vi "Load Settings from XML.vi"(8 "error in (no error)":errorcluster, 11 "Settings in":T1={"Logging Configuration"={"Log File Base Path"=path "", "NbrIma"=1}, "camera"={"Camera.lvclass"=refnum, "InClusTiming 2"={"Pixelclock"=24, "Exposure"=46.39115, "ExposureTimeBase"=2, "Framerate"=14.99615, "TriggerMode"=0}, "ROI"={"PosX"=0, "PosY"=0, "Width"=0, "Height"=0}, "File Path Control"=path "", "mirror.lvclass"=refnum}} {"camera"."InClusTiming 2"."TriggerMode" items=["Auto", "Software", "External sequence start ", "External exposure control"]; "camera"."InClusTiming 2"."ExposureTimeBase" items=["nanoseconds", "microseconds", "milliseconds"]; "camera"."InClusTiming 2"."Pixelclock" min=1 max=400 step=1 scale=0.05915..400.0 scale format="%#.3g"; "camera"."InClusTiming 2"."Framerate" min=0.05915 max=2000.0 step=1.0 scale=0.05915..100.0 scale format="%#.3g"; "camera"."InClusTiming 2"."Exposure" min=0.05915 max=2000.0 step=1.0 scale=0.05915..100.0 scale format="%#.3g"; "Logging Configuration"."NbrIma" min=1 step=1}) -> (0 "error out":errorcluster, 3 "Settings out":T1={"Logging Configuration"={"Log File Base Path"=path "", "NbrIma"=1}, "camera"={"Camera.lvclass"=refnum, "InClusTiming 2"={"Pixelclock"=24, "Exposure"=46.39115, "ExposureTimeBase"=2, "Framerate"=14.99615, "TriggerMode"=0}, "ROI"={"PosX"=0, "PosY"=0, "Width"=0, "Height"=0}, "File Path Control"=path "", "mirror.lvclass"=refnum}} {"camera"."InClusTiming 2"."TriggerMode" items=["Auto", "Software", "External sequence start ", "External exposure control"]; "camera"."InClusTiming 2"."ExposureTimeBase" items=["nanoseconds", "microseconds", "milliseconds"]; "camera"."InClusTiming 2"."Pixelclock" min=1 max=400 step=1 scale=0.05915..400.0 scale format="%#.3g"; "camera"."InClusTiming 2"."Framerate" min=0.05915 max=2000.0 step=1.0 scale=0.05915..100.0 scale format="%#.3g"; "camera"."InClusTiming 2"."Exposure" min=0.05915 max=2000.0 step=1.0 scale=0.05915..100.0 scale format="%#.3g"; "Logging Configuration"."NbrIma" min=1 step=1})   [LabVIEW 2020, in "Settings.lvlib"]
doc: "Attempts to load previous user specified settings from an XML file.\n\nThis VI will not generate an error. If a suitable XML file can't be loaded and parsed then it will simply return the default settings."
uses:
  Settings.lvlib
  Settings.ctl
  CLASS/Image Acquisition Class/Camera.lvclass
  MIRROR/mirror.lvclass
  LOGGING/Logging Configuration.ctl
  ACQUISITION/HardwareConfiguration.ctl
  <vilib>/Utility/xml.llb/Read From XML File(string).vi
  <vilib>/Utility/xml.llb/Write to XML File(string).vi
  LOGGING/Logging.lvlib
  ACQUISITION/Acquisition.lvlib
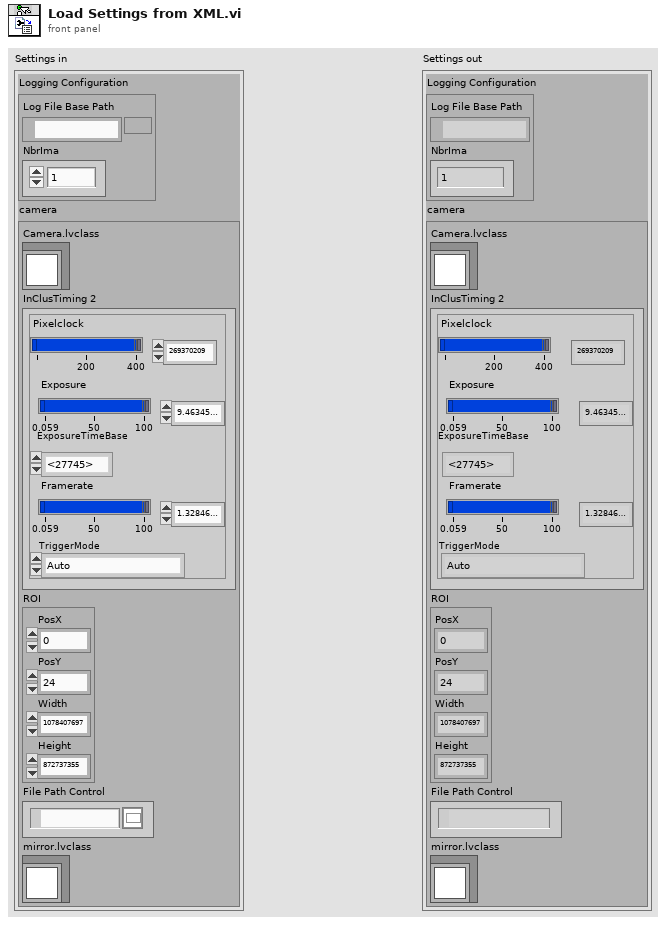
[diagram p1: front panel]
types:
  T1 = typedef "Settings.lvlib/Settings.ctl" = cluster{"Logging Configuration":T2, "camera":T3}
  T2 = typedef "Logging.lvlib/Logging Configuration.ctl" = cluster{"Log File Base Path":path, "NbrIma":i32}
  T3 = typedef "Acquisition.lvlib/HardwareConfiguration.ctl" = cluster{"Camera.lvclass":refnum<class "Camera.lvclass">, "InClusTiming 2":cluster{"Pixelclock":i32, "Exposure":dbl, "ExposureTimeBase":u16, "Framerate":dbl, "TriggerMode":u16}, "ROI":cluster{"PosX":i32, "PosY":i32, "Width":i32, "Height":i32}, "File Path Control":path, "mirror.lvclass":refnum<class "mirror.lvclass">}
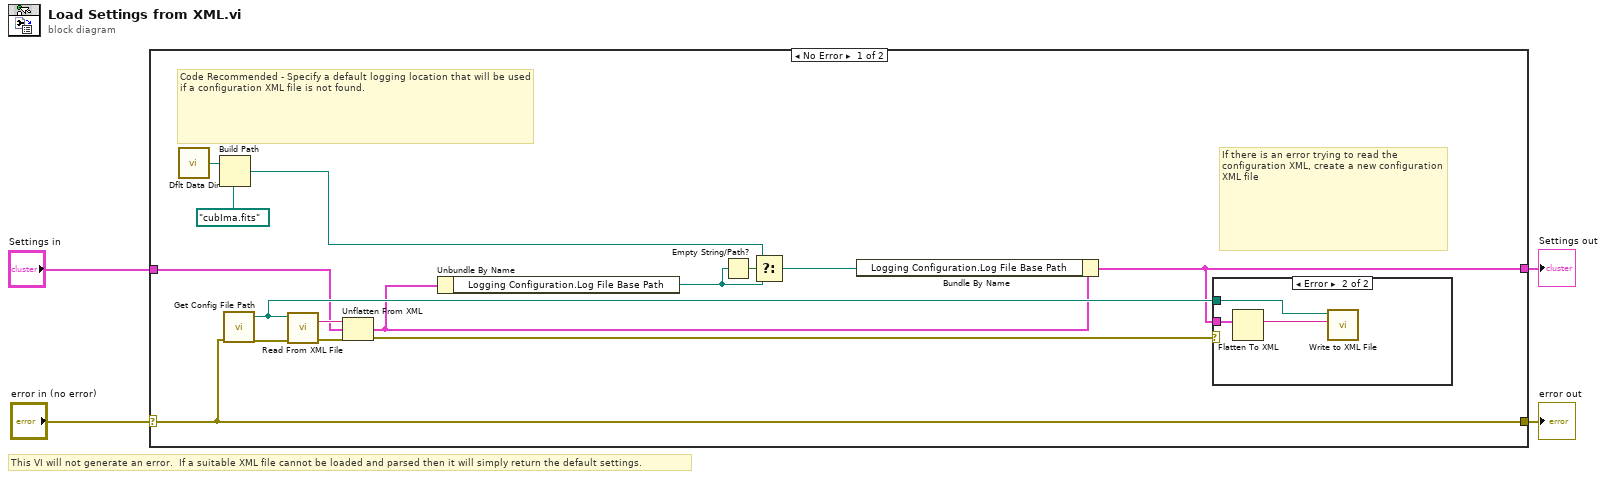
[diagram p0: block diagram]
diagram:
  # "This VI will not generate an error.  If a suitable XML file cannot be loaded and parsed then it will simply return the default settings."
  n1 = case shown="No Error" "error in (no error)" {
    selector: "error in (no error)" -> [w17 w24]
    tunnel: [w17 w24] -> w3
    tunnel: "Settings in" -> [w11 w23]
    tunnel: [w5 w23] -> w1
    frame No Error {
      # "If there is an error trying to read the configuration XML, create a new configuration XML file"
      # "Code Recommended - Specify a default logging location that will be used if a configuration XML file is not found."
      n2 = call <vilib>:"Dflt Data Dir.vi"() -> ("App:Default Data Directory"=w16:path)
      n3 = Build Path(base path=w16, name or relative path=path "cubIma.fits" ("App:Default Data Directory")) -> (appended path=w8:path)
      n4 = call "Get Config File Path.vi"("error in (no error)"=w17) -> ("error out"=w19:errorcluster, "XML File Path"=w14:path)  [unwired: 9 in]
      n5 = call-poly <vilib>:"Read From XML File.vi"("error in (no error)"=w19, "XML File Path"=w14) -> ("error out"=w13:errorcluster, "XML Elements"=w18:string)  [unwired: 7 in, 1 out]
      n6 = Unflatten From XML(xml string=w18, type=w11, error in (no error)=w13) -> (value=w7:T1, error out=w12:errorcluster)
      n7 = Unbundle By Name(w7) -> ("Logging Configuration.Log File Base Path"=w9:path)
      n8 = Empty String/Path?(string/path=w9) -> (empty?=w10:bool)
      n9 = Select(t=w8, s=w10, f=w9) -> (s? t:f=w6:path)
      n10 = Bundle By Name(cluster=w7, "Logging Configuration.Log File Base Path"=w6) -> (w5:T1)
      n11 = case shown="Error" w12 {
        tunnel: w5 -> [_ w22]
        tunnel: w14 -> [_ w20]
        frame No Error {
        }
        frame Error {
          n12 = Flatten To XML(6:w22) -> (2:w21:string)
          n13 = call-poly <vilib>:"Write to XML File.vi"("XML Input"=w21, "XML File Path"=w20) -> ()  [unwired: 7 in, 3 out]
        }
      }
    }
    frame Error {
    }
  }
  "error out" <- w3
  "Settings out" <- w1
